vi "networkstream_test_PC.vi"() -> ()   [LabVIEW 2017]
panel:
  in  "stop":bool
  out "data out":dbl
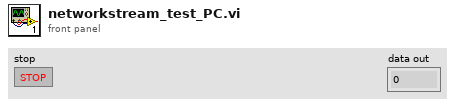
[diagram p1: front panel]
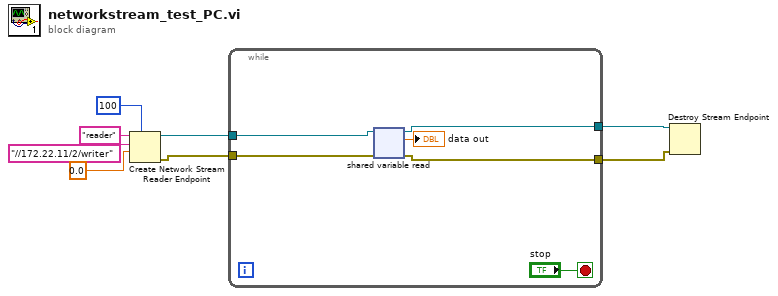
[diagram p0: block diagram]
diagram:
  n1 = Create Network Stream Reader Endpoint(7:100 ("reader buffer size"), 9:0.0, 10:"//172.22.11/2/writer" ("writer url"), 11:"reader" ("reader name")) -> (0:w4:errorcluster, 3:w5:refnum<k21>)  [unwired: 3 in]
  n2 = while {
    tunnel: w5 -> [w14]
    tunnel: w4 -> [w13]
    tunnel: [w11] -> w3
    tunnel: [w10] -> w2
    stop <- "stop" stop-if-true
    n3 = shared-variable-read(w14, w13) -> (w11:refnum<k21>, w10:errorcluster, →"data out":dbl)  [unwired: 1 in, 1 out]
  }
  n4 = Destroy Stream Endpoint(8:w2, 11:w3) -> ()  [unwired: 1 out]
